vi "Magnet Set Field (Manual).vi"(6 "Field Strength":dbl, 7 "Polarity":bool, 8 "error in (no error)":errorcluster, 11 "VISA resource name in":refnum<visa-resource-name>) -> (0 "error out":errorcluster, 3 "VISA resource name out":refnum<visa-resource-name>)   [LabVIEW 2016, in "Hall Effect Library.lvlib"]
uses:
  Hall Effect Library.lvlib
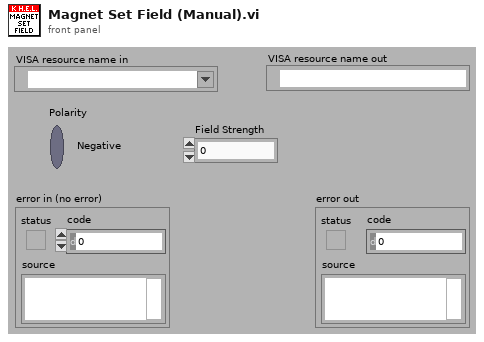
[diagram p1: front panel]
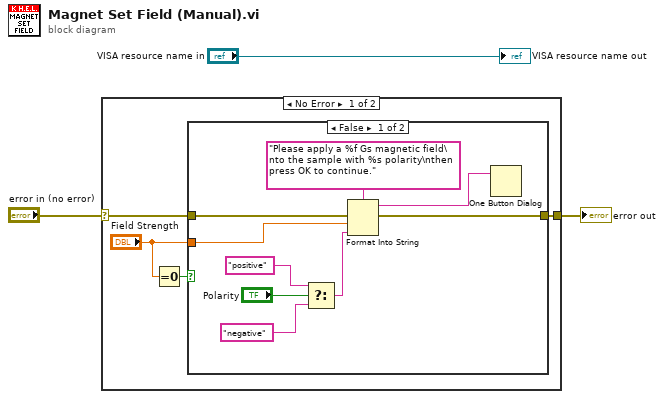
[diagram p0: block diagram]
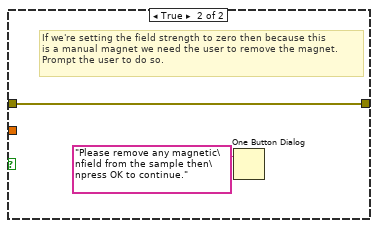
[diagram p2: hidden frame]
diagram:
  n1 = case shown="No Error" "error in (no error)" {
    selector: "error in (no error)" -> [w4 w19]
    tunnel: [w7 w19] -> w2
    frame No Error {
      n2 = Equal To 0?(x="Field Strength") -> (x = 0?=w6:bool)
      n3 = case shown="False" w6 {
        tunnel: w4 -> [w11 w17]
        tunnel: [w10 w17] -> w7
        tunnel: "Field Strength" -> [w8 _]
        frame False {
          n4 = Select(t="positive", s="Polarity", f="negative") -> (s? t:f=w9:string)
          n5 = Format Into String(format string="Please apply a %f Gs magnetic field\nto the sample with %s polarity\nthen press OK to continue." ("message"), error in=w11, w8, w9) -> (resulting string=w12:string, error out=w10:errorcluster)  [unwired: 1 in]
          n6 = One Button Dialog(message=w12) -> ()  [unwired: 2 out]
        }
        frame True {
          # "If we're setting the field strength to zero then because this\nis a manual magnet we need the user to remove the magnet.\nPrompt the user to do so."
          n7 = One Button Dialog(message="Please remove any magnetic\nfield from the sample then\npress OK to continue.") -> ()  [unwired: 2 out]
        }
      }
    }
    frame Error {
    }
  }
  "error out" <- w2
  "VISA resource name out" <- "VISA resource name in"
